vi "GUILib.application example main.vi"() -> ()   [LabVIEW 2012, in "GUILib.lvlib"]
doc: "This is an example of basic GUI.\n\ndescriptionHelpStart\nThis is a GUI for the XY facility. Bla bla bla...\ndescriptionHelpStop\n\naboutHelpStart\nXY GUI by author\nCopyright\nGPL\naboutHelpStop\n\nmenuHelpStart\nexplain menu here...\nmenuHelpStop"
uses:
  GUILib.lvlib
  GUILib.userEventsMainType.ctl
  UtilityLib/UtilityLib.valueStatus.ctl
  UtilityLib/UtilityLib.helpType.ctl
  UtilityLib/UtilityLib.lvlib
panel:
  out "infoStatus4":string
  out "infoStatus3":string
  out "infoStatus2":string
  out "additionalInfo":string
  out "versionInfo":string
  out "facilityName":string
  out "mainSystemName":string
  out "actSystemState":string
  out "mainSystemState":string
  out "actualSystemName":string
  out "timeAndDate":string
  in  "userEventsMain":T1
  in  "topSystem":bool
  in  "userEventsMainType":T1
  # "information (program name, experiment, facility, version, user, ...)"
  # "messages, warnings, errors, ...."
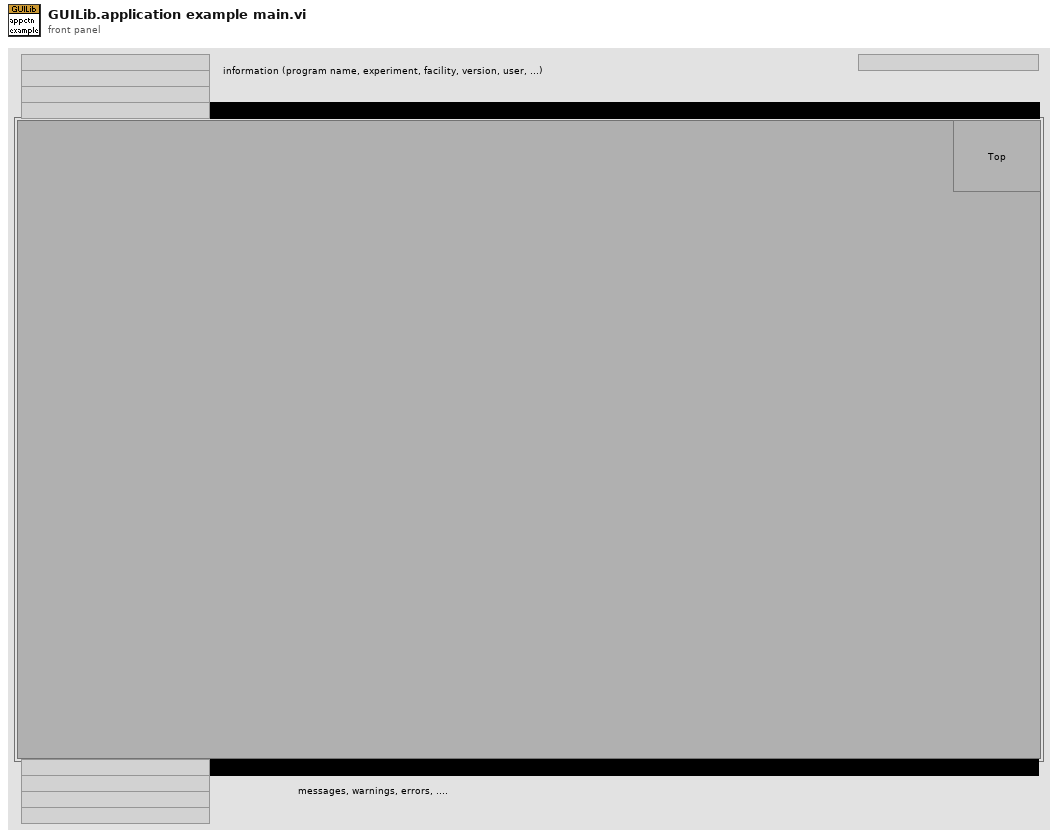
[diagram p1: front panel]
types:
  T1 = typedef "GUILib.lvlib/GUILib.userEventsMainType.ctl" = cluster{"data":string, "dataType":i32}
  T2 = typedef "UtilityLib.lvlib/UtilityLib.helpType.ctl" = enum16{"unknown", "menu", "description", "about", "special0", "special1", "special2"}
  T3 = typedef "UtilityLib.lvlib/UtilityLib.valueStatus.ctl" = enum16{"no info available", "stand by/off", "on", "warning", "alarm/malfunction", "not implemented", "user action required", "important information", "system default", "control default", "indicator default", "button default"}
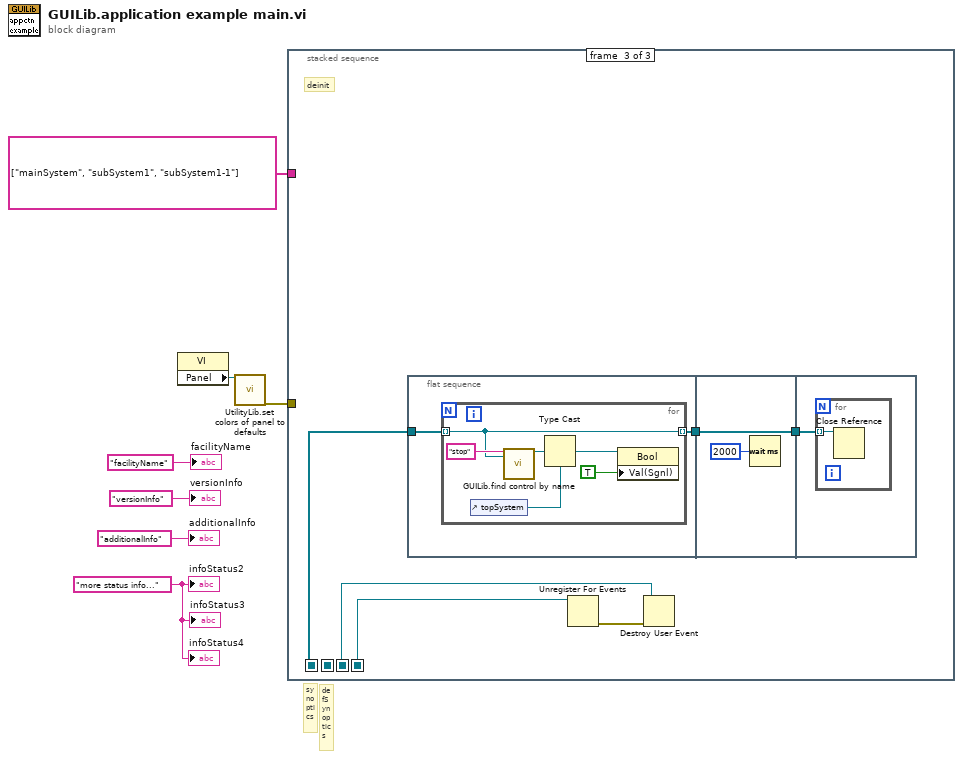
[diagram p0: block diagram]
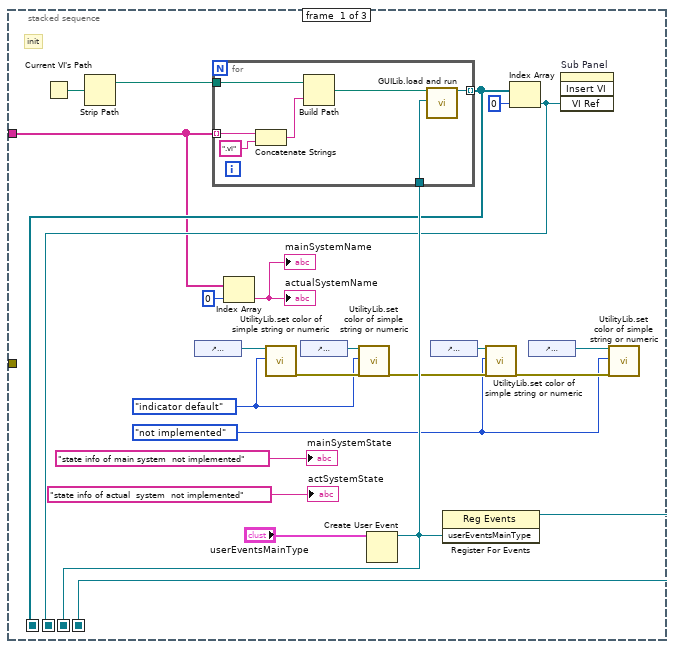
[diagram p2: hidden frame]
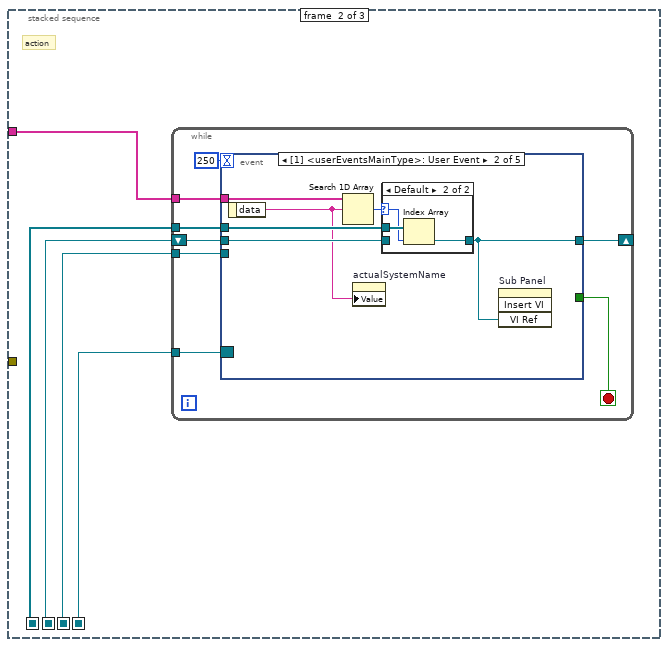
[diagram p3: hidden frame]
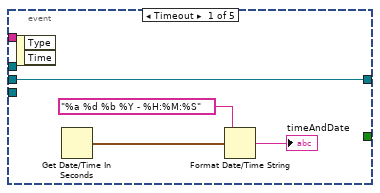
[diagram p4: hidden frame]
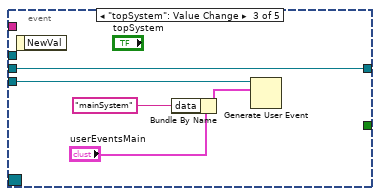
[diagram p6: hidden frame]
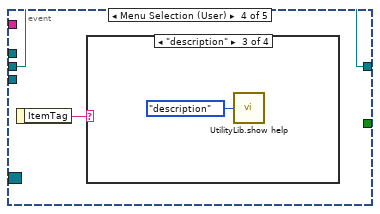
[diagram p7: hidden frame]
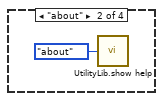
[diagram p9: hidden frame]
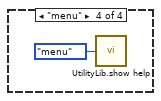
[diagram p10: hidden frame]
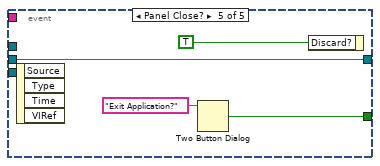
[diagram p11: hidden frame]
diagram:
  w1 = "more status info..." ("info1")
  # "defSynoptics"
  # "synoptics"
  n1 = property on="Property Node" class="VI"() -> ("Panel"=w6:refnum<vi>)  [unwired: 2 in, 2 out]
  n2 = call "UtilityLib.set colors of panel to defaults.vi"("Front Panel"=w6) -> ("error out"=w5:errorcluster)  [unwired: 18 in]
  n3 = stacked-sequence {
    seq-local: [w25 _ _] -> [_ w38 w78]
    seq-local: [w28 _ _] -> [_ w41 w83]
    seq-local: [w26 _ _] -> [_ w37 w81]
    seq-local: [w22 _ _] -> [_ w40 _]
    tunnel: string[] ["mainSystem", "subSystem1", "subSystem1-1"] -> [w20 w39 _]
    tunnel: w5 -> [_ _ _]
    frame #0 {
      w9 = UtilityLib.valueStatus."not implemented" ("valueStatus")
      w16 = UtilityLib.valueStatus."indicator default" ("valueStatus")
      # "init"
      n4 = Current VI's Path() -> (path=w29:path)
      n5 = Strip Path(path=w29) -> (stripped path=w23:path)  [unwired: 1 out]
      n6 = control-ref of="timeAndDate"() -> (w19:refnum<vi>)
      n7 = Index Array(array=w20, index=0) -> (element=→"actualSystemName" →"mainSystemName":string)
      n8 = call "UtilityLib.set color of simple string or numeric.vi"("simpleString"=w19, "valueStatus"=w16) -> ("error out"=w17:errorcluster)  [unwired: 17 in]
      n9 = control-ref of="actualSystemName"() -> (w18:refnum<vi>)
      n10 = call "UtilityLib.set color of simple string or numeric.vi"("simpleString"=w18, "valueStatus"=w16, "error in (no error)"=w17) -> ("error out"=w13:errorcluster)  [unwired: 16 in]
      n11 = Create User Event(user event datatype="userEventsMainType") -> (user event=w26:refnum<user-event>)  [unwired: 1 in, 1 out]
      n12 = for {
        tunnel: [w35] -> w25 mode=indexing
        tunnel: w26 -> [w34]
        tunnel: w20 -> [w33] mode=indexing
        tunnel: w23 -> [w32]
        n13 = Concatenate Strings(w33, ".vi" ("string")) -> (w31:string)
        n14 = Build Path(base path=w32, name or relative path=w31) -> (appended path=w36:path)
        n15 = call "GUILib.load and run.vi"("path"=w36, "userEvent"=w34) -> ("VIRef"=w35:refnum<vi>)  [unwired: 16 in, 1 out]
      }
      n16 = control-ref of="mainSystemState"() -> (w14:refnum<vi>)
      n17 = register-events(w26) -> (reference out=w28:refnum<event-registration>)  [unwired: 2 in, 1 out]
      n18 = call "UtilityLib.set color of simple string or numeric.vi"("simpleString"=w14, "valueStatus"=w9, "error in (no error)"=w13) -> ("error out"=w10:errorcluster)  [unwired: 16 in]
      n19 = Index Array(array=w25, index=0) -> (element=w22:refnum<vi>)
      n20 = control-ref of="actSystemState"() -> (w11:refnum<vi>)
      n21 = invoke on="Sub Panel" class="SubPnl" method="Insert VI"("VI Ref"=w22) -> ()  [unwired: 3 in, 4 out]
      n22 = call "UtilityLib.set color of simple string or numeric.vi"("simpleString"=w11, "valueStatus"=w9, "error in (no error)"=w10) -> ()  [unwired: 16 in, 1 out]
      "mainSystemState" <- "state info of main system  not implemented" ("systemState")
      "actSystemState" <- "state info of actual  system  not implemented" ("systemState")
    }
    frame #1 {
      # "action"
      n23 = while {
        tunnel: w41 -> [w48]
        shift-right: [w47] -> _
        shift-left: w40 -> [w46]
        tunnel: w39 -> [w45]
        tunnel: w38 -> [w44]
        tunnel: w37 -> [w43]
        stop <- w49 stop-if-true
        n24 = event shown="[1] <userEventsMainType>: User Event" {
          selector: w48 -> [_ _ _ _ _]
          dyn-events: _ -> [_ _ _ _ _]
          timeout: 250 -> [_ _ _ _ _]
          tunnel: [_ _ _ _ w75] -> w49
          tunnel: [w53 w55 w68 w70 w74] -> w47
          tunnel: w46 -> [w53 w59 w68 w70 w74]
          tunnel: w45 -> [_ w58 _ _ _]
          tunnel: w44 -> [_ w56 _ _ _]
          tunnel: w43 -> [_ _ w67 _ _]
          event Timeout {
            n25 = event-data() -> ()  [unwired: 1 in, 2 out]
            n26 = Get Date/Time In Seconds() -> (seconds since 1Jan1904=w52:timestamp)
            n27 = Format Date/Time String(time format string (%c)="%a %d %b %Y - %H:%M:%S", seconds (now)=w52) -> (date/time string=→"timeAndDate":string)  [unwired: 1 in]
          }
          event User Event {
            n28 = event-data() -> ("data"=w54:string)  [unwired: 1 in]
            n29 = Search 1D Array(1D array=w58, element=w54) -> (index of element=w57:i32)  [unwired: 1 in]
            n30 = property on="actualSystemName" class="Str"("Value"=w54) -> ()  [unwired: 2 in, 2 out]
            n31 = case shown="Default" w57 {
              selector: w57 -> [_ w62]
              tunnel: [w60 w61] -> w55
              tunnel: w59 -> [w60 _]
              tunnel: w56 -> [_ w63]
              frame -1 {
              }
              frame Default {
                n32 = Index Array(array=w63, index=w62) -> (element=w61:refnum<vi>)
              }
            }
            n33 = invoke on="Sub Panel" class="SubPnl" method="Insert VI"("VI Ref"=w55) -> ()  [unwired: 3 in, 4 out]
          }
          event "topSystem": Value Change {
            n34 = event-data() -> ()  [unwired: 1 in, 1 out]
            n35 = Bundle By Name(cluster="userEventsMain", "data"="mainSystem" ("systemToShow")) -> (w66:T1)
            n36 = Generate User Event(user event=w67, event data cluster=w66) -> ()  [unwired: 1 in, 2 out]
          }
          event Menu Selection (User) {
            n37 = event-data() -> ("ItemTag"=w69:string)  [unwired: 1 in]
            n38 = case shown="\"description\"" w69 {
              frame "False", Default {
              }
              frame "about" {
                n39 = call "UtilityLib.show help.vi"("helpType"=UtilityLib.helpType."about") -> ()
              }
              frame "description" {
                n40 = call "UtilityLib.show help.vi"("helpType"=UtilityLib.helpType."description") -> ()
              }
              frame "menu" {
                n41 = call "UtilityLib.show help.vi"("helpType"=UtilityLib.helpType."menu") -> ()
              }
            }
          }
          event Panel Close? {
            n42 = event-data() -> ()  [unwired: 1 in, 4 out]
            n43 = Two Button Dialog(message="Exit Application?") -> (T button?=w75:bool)  [unwired: 2 in]
            n44 = event-data ("Event Filter Node")("Discard?"=TRUE) -> ()  [unwired: 1 in, 1 out]
          }
        }
      }
    }
    frame #2 {
      # "deinit"
      n45 = flat-sequence {
        tunnel: [w85] -> w80
        tunnel: w78 -> [w84]
        tunnel: w80 -> [w92]
        tunnel: [w92] -> w79
        tunnel: w79 -> [w94]
        frame #0 {
          n46 = for {
            tunnel: [w90] -> w85 mode=indexing
            tunnel: w84 -> [w90] mode=indexing
            n47 = control-ref of="topSystem"() -> (w87:refnum<vi>)
            n48 = call "GUILib.find control by name.vi"("control name"="stop", "VIRef"=w90) -> ("controlRef"=w89:refnum<vi>)  [unwired: 16 in, 1 out]
            n49 = Type Cast(type=w87, x=w89) -> (*(type *) &x=w88:refnum<vi>)
            n50 = property on="Property Node" class="Bool"(reference=w88, "Val(Sgnl)"=TRUE) -> ()  [unwired: 1 in, 2 out]
          }
        }
        frame #1 {
          n51 = Wait (ms)(milliseconds to wait=u32 2000) -> ()  [unwired: 1 out]
        }
        frame #2 {
          n52 = for {
            tunnel: w94 -> [w95] mode=indexing
            n53 = Close Reference(reference=w95) -> ()  [unwired: 1 in, 1 out]
          }
        }
      }
      n54 = Unregister For Events(event registration refnum=w83) -> (error out=w82:errorcluster)  [unwired: 1 in]
      n55 = Destroy User Event(user event=w81, error in=w82) -> ()  [unwired: 1 out]
    }
  }
  "facilityName" <- "facilityName" ("facilityName")
  "versionInfo" <- "versionInfo" ("actualSystemName 3")
  "additionalInfo" <- "additionalInfo" ("additionalInfo")
  "infoStatus2" <- w1
  "infoStatus3" <- w1
  "infoStatus4" <- w1
